vi "FanSpeedControl.vi"() -> ()   [LabVIEW 2018]
uses:
  C:/Users/Public/Documents/Photometrics/PMQI-LabViewSamples/Examples/Dependencies/PVCamNET.dll
  Public/Documents/Photometrics/PMQI-LabViewSamples/Examples/Dependencies/PVCamNET.dll
panel:
  in  "?":bool
  out "Current Value":string
  in  "Fan Speed":string(combo)
  in  "?":bool
  in  "?":bool
  # "FanSpeedControl.vi\n\nDescription:\nThis sample code lets the user control the fan speed. \n\nSteps to run:\n1. Click \"Run\"\n2. Click \"START\"\n2. Select Fan Speed\n3. Click \"Set Fan Speed\"\n4. Click \"STOP\""
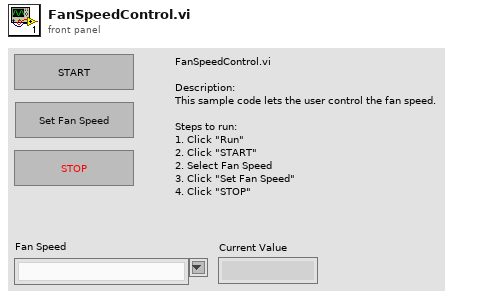
[diagram p1: front panel]
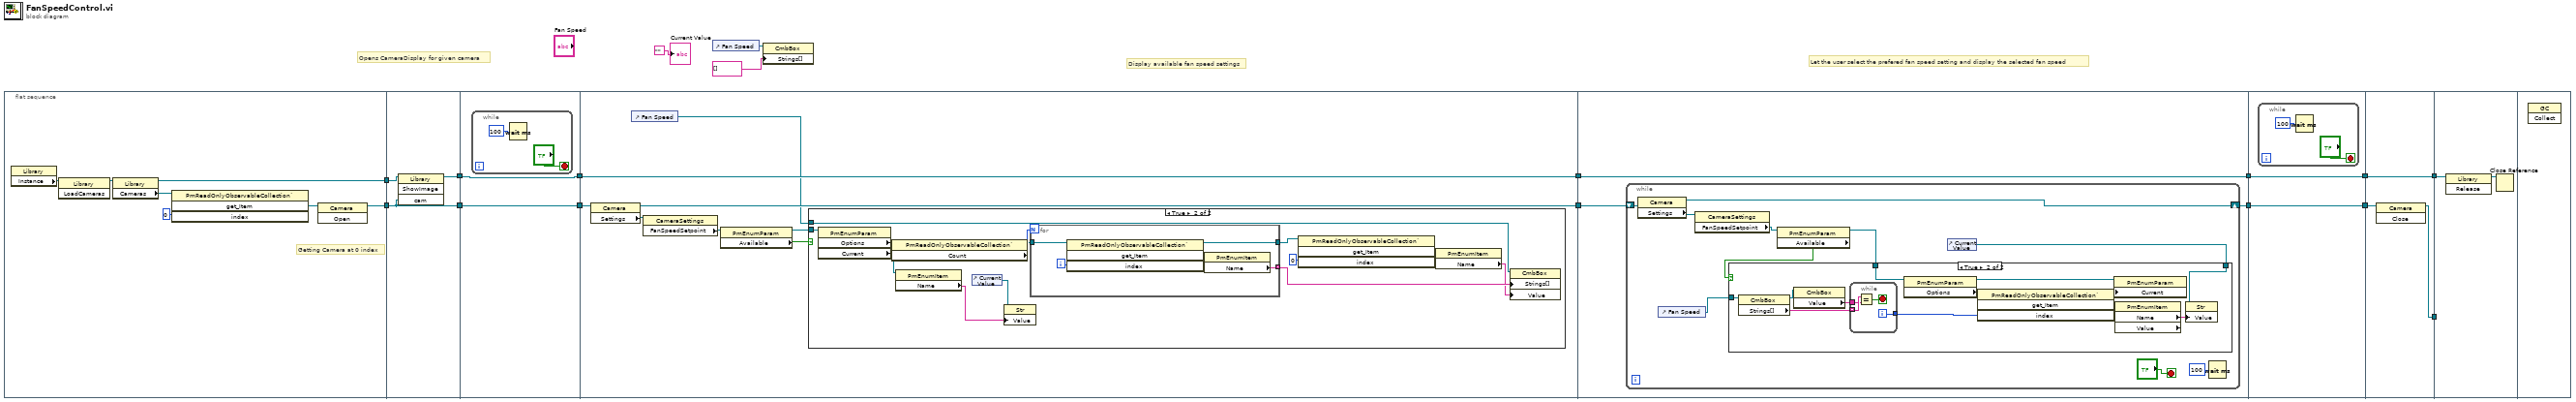
[diagram p0: block diagram]
diagram:
  # "Let the user select the prefered fan speed setting and display the selected fan speed"
  # "Display available fan speed settings"
  # "Opens CameraDisplay for given camera"
  n1 = flat-sequence {
    tunnel: [w20] -> w17
    tunnel: [w21] -> w16
    tunnel: w17 -> [w27]
    tunnel: w16 -> [w26]
    tunnel: [w26] -> w15
    tunnel: [w25] -> w14
    tunnel: w15 -> [w29]
    tunnel: [w29] -> w12
    tunnel: w14 -> [w28]
    tunnel: [w28] -> w13
    tunnel: [w39] -> w7
    tunnel: [w38] -> w5
    tunnel: w13 -> [w38]
    tunnel: w12 -> [w37]
    tunnel: w7 -> [w60]
    tunnel: [w58] -> w6
    tunnel: w5 -> [w59]
    tunnel: [w59] -> w4
    tunnel: w6 -> [w87]
    tunnel: [w87] -> w9
    tunnel: [w86] -> w8
    tunnel: w4 -> [w86]
    tunnel: w9 -> [w92]
    tunnel: w8 -> [w90]
    tunnel: [w91] -> w11
    tunnel: [w90] -> w10
    tunnel: w11 -> [_]
    tunnel: w10 -> [w94]
    frame #0 {
      # "Getting Camera at 0 index"
      n2 = property class="Library"() -> ("Instance"=w19:refnum<k24>)  [unwired: 2 in, 2 out]
      n3 = invoke class="Library" method="LoadCameras"(reference=w19) -> (reference out=w18:refnum<k24>)  [unwired: 2 in, 2 out]
      n4 = property class="Library"(reference=w18) -> (reference out=w20:refnum<k24>, "Cameras"=w24:refnum<k24>)  [unwired: 1 in, 1 out]
      n5 = invoke class="PmReadOnlyObservableCollection`" method="get_Item"(reference=w24, "index"=0) -> ("get_Item"=w22:refnum<k24>)  [unwired: 2 in, 3 out]
      n6 = invoke class="Camera" method="Open"(reference=w22) -> (reference out=w21:refnum<k24>)  [unwired: 2 in, 2 out]
    }
    frame #1 {
      n7 = invoke class="Library" method="ShowImage"(reference=w27, "cam"=w26) -> (reference out=w25:refnum<k24>)  [unwired: 2 in, 3 out]
    }
    frame #2 {
      n8 = while {
        stop <- "?" stop-if-true
        n9 = Wait (ms)(milliseconds to wait=u32 100) -> ()  [unwired: 1 out]
      }
    }
    frame #3 {
      n10 = property class="Camera"(reference=w37) -> (reference out=w39:refnum<k24>, "Settings"=w36:refnum<k24>)  [unwired: 1 in, 1 out]
      n11 = control-ref of="Fan Speed"() -> (w32:refnum<vi>)
      n12 = property class="CameraSettings"(reference=w36) -> ("FanSpeedSetpoint"=w35:refnum<k24>)  [unwired: 1 in, 2 out]
      n13 = property class="PmEnumParam"(reference=w35) -> (reference out=w33:refnum<k24>, "Available"=w34:bool)  [unwired: 1 in, 1 out]
      n14 = case shown="True" w34 {
        tunnel: w32 -> [_ w44]
        tunnel: w33 -> [_ w43]
        frame False {
        }
        frame True {
          n15 = property class="PmEnumParam"(reference=w43) -> ("Options"=w52:refnum<k24>, "Current"=w42:refnum<k24>)  [unwired: 1 in, 2 out]
          n16 = property class="PmReadOnlyObservableCollection`"(reference=w52) -> (reference out=w50:refnum<k24>, "Count"=w51:i32)  [unwired: 1 in, 1 out]
          n17 = property class="PmEnumItem"(reference=w42) -> ("Name"=w40:string)  [unwired: 1 in, 2 out]
          n18 = control-ref of="Current Value"() -> (w41:refnum<vi>)
          n19 = property class="Str"(reference=w41, "Value"=w40) -> ()  [unwired: 1 in, 2 out]
          n20 = for {
            N: w51 -> [_]
            tunnel: w50 -> [w57]
            tunnel: [w54] -> w48
            tunnel: [w53] -> w49 mode=indexing
            i -> [w56]
            n21 = invoke class="PmReadOnlyObservableCollection`" method="get_Item"(reference=w57, "index"=w56) -> (reference out=w54:refnum<k24>, "get_Item"=w55:refnum<k24>)  [unwired: 2 in, 2 out]
            n22 = property class="PmEnumItem"(reference=w55) -> ("Name"=w53:string)  [unwired: 1 in, 2 out]
          }
          n23 = invoke class="PmReadOnlyObservableCollection`" method="get_Item"(reference=w48, "index"=0) -> ("get_Item"=w46:refnum<k24>)  [unwired: 2 in, 3 out]
          n24 = property class="PmEnumItem"(reference=w46) -> ("Name"=w45:string)  [unwired: 1 in, 2 out]
          n25 = property class="CmbBox"(reference=w44, "Strings[]"=w49, "Value"=w45) -> ()  [unwired: 1 in, 2 out]
        }
      }
    }
    frame #4 {
      n26 = while {
        shift-right: [w63] -> w58
        shift-left: w60 -> [w69]
        stop <- "?" stop-if-true
        n27 = property class="Camera"(reference=w69) -> (reference out=w63:refnum<k24>, "Settings"=w70:refnum<k24>)  [unwired: 1 in, 1 out]
        n28 = control-ref of="Fan Speed"() -> (w65:refnum<vi>)
        n29 = property class="CameraSettings"(reference=w70) -> ("FanSpeedSetpoint"=w68:refnum<k24>)  [unwired: 1 in, 2 out]
        n30 = property class="PmEnumParam"(reference=w68) -> (reference out=w66:refnum<k24>, "Available"=w67:bool)  [unwired: 1 in, 1 out]
        n31 = control-ref of="Current Value"() -> (w64:refnum<vi>)
        n32 = case shown="True" w67 {
          tunnel: w66 -> [_ w80]
          tunnel: w65 -> [_ w76]
          tunnel: w64 -> [_ w73]
          frame False {
          }
          frame True {
            n33 = property class="CmbBox"(reference=w76) -> (reference out=w75:refnum<vi>, "Strings[]"=w81:string[])  [unwired: 1 in, 1 out]
            n34 = property class="CmbBox"(reference=w75) -> ("Value"=w74:string)  [unwired: 1 in, 2 out]
            n35 = while {
              tunnel: w81 -> [w85] mode=indexing
              tunnel: [w83] -> w78
              tunnel: w74 -> [w82]
              i -> [w83]
              stop <- w84 stop-if-true
              n36 = Equal?(x=w85, y=w82) -> (x = y?=w84:bool)
            }
            n37 = property class="PmEnumParam"(reference=w80) -> (reference out=w77:refnum<k24>, "Options"=w79:refnum<k24>)  [unwired: 1 in, 1 out]
            n38 = invoke class="PmReadOnlyObservableCollection`" method="get_Item"(reference=w79, "index"=w78) -> ("get_Item"=w71:refnum<k24>)  [unwired: 2 in, 3 out]
            n39 = property class="PmEnumParam"(reference=w77, "Current"=w71) -> ()  [unwired: 1 in, 2 out]
            n40 = property class="PmEnumItem" props=["Name", "Value"](reference=w71) -> ("Name"=w72:string)  [unwired: 1 in, 3 out]
            n41 = property class="Str"(reference=w73, "Value"=w72) -> ()  [unwired: 1 in, 2 out]
          }
        }
        n42 = Wait (ms)(milliseconds to wait=u32 100) -> ()  [unwired: 1 out]
      }
    }
    frame #5 {
      n43 = while {
        stop <- "?" stop-if-true
        n44 = Wait (ms)(milliseconds to wait=u32 100) -> ()  [unwired: 1 out]
      }
    }
    frame #6 {
      n45 = invoke class="Camera" method="Close"(reference=w92) -> (reference out=w91:refnum<k24>)  [unwired: 2 in, 2 out]
    }
    frame #7 {
      n46 = invoke class="Library" method="Release"(reference=w94) -> (reference out=w93:refnum<k24>)  [unwired: 2 in, 2 out]
      n47 = Close Reference(reference=w93) -> ()  [unwired: 1 in, 1 out]
    }
    frame #8 {
      n48 = invoke class="GC" method="Collect"() -> ()  [unwired: 3 in, 3 out]
    }
  }
  n49 = control-ref of="Fan Speed"() -> (w2:refnum<vi>)
  n50 = property class="CmbBox"(reference=w2, "Strings[]"=string[] [] ("Strings []")) -> ()  [unwired: 1 in, 2 out]
  "Current Value" <- ""
